vi "RichToFlatnixnet_grpc_DbGetDBCAttributeSizeResponse.vi"(5 "OutputClusterType":T1, 11 "InputCluster":T2) -> (3 "OutputCluster":T1)   [LabVIEW 2025, in "grpc-xnet_client.lvlib"]
uses:
  nixnet_grpc_DbGetDBCAttributeSizeResponse.ctl
  nixnet_grpc_DbGetDBCAttributeSizeResponse_Flat.ctl
  grpc-xnet_client.lvlib
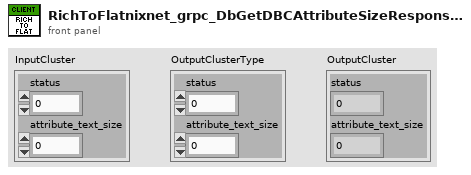
[diagram p1: front panel]
types:
  T1 = typedef "grpc-xnet_client.lvlib/nixnet_grpc_DbGetDBCAttributeSizeResponse_Flat.ctl" = cluster{"status":i32, "attribute_text_size":u32}
  T2 = typedef "grpc-xnet_client.lvlib/nixnet_grpc_DbGetDBCAttributeSizeResponse.ctl" = cluster{"status":i32, "attribute_text_size":u32}
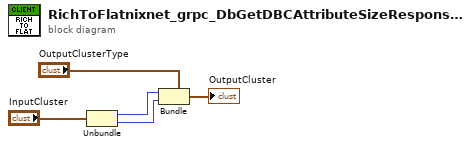
[diagram p0: block diagram]
diagram:
  n1 = Unbundle "Unbundle"("InputCluster") -> ("status"=w2:i32, "attribute_text_size"=w1:u32)
  n2 = Bundle "Bundle"(cluster="OutputClusterType", "status"=w2, "attribute_text_size"=w1) -> (→"OutputCluster":T1)
